vi "Scale.vi"(8 "error in (no error)":errorcluster, 10 "Scale Factor":dbl, 11 "Point in":refnum<class "PointSpecialized.lvclass">) -> (0 "error out":errorcluster, 3 "Point out":refnum<class "PointSpecialized.lvclass">)   [LabVIEW 2021, in "Picture2D.lvlib" / "PointSpecialized.lvclass"]
uses:
  PointSpecialized.lvclass
  PointSpecialized.lvclass/PointSpecialized.ctl
  Pen/Pen.lvclass
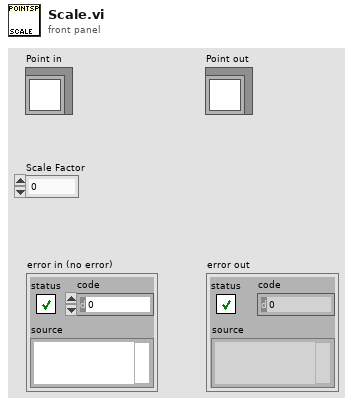
[diagram p1: front panel]
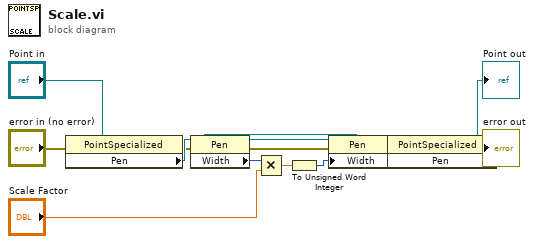
[diagram p0: block diagram]
diagram:
  n1 = property class="PointSpecialized"(reference="Point in", error in="error in (no error)") -> (reference out=w7:refnum<class "PointSpecialized.lvclass">, error out=w5:errorcluster, "Pen"=w15:refnum<class "Pen.lvclass">)
  n2 = property class="Pen"(reference=w15, error in=w5) -> (reference out=w14:refnum<class "Pen.lvclass">, error out=w4:errorcluster, "Width"=w11:u16)
  n3 = Multiply(x=w11, y="Scale Factor") -> (x*y=w10:dbl)
  n4 = To Unsigned Word Integer(number=w10) -> (unsigned 16bit integer=w9:u16)
  n5 = property class="Pen"(reference=w14, error in=w4, "Width"=w9) -> (reference out=w13:refnum<class "Pen.lvclass">, error out=w3:errorcluster)
  n6 = property class="PointSpecialized"(reference=w7, error in=w3, "Pen"=w13) -> (reference out=→"Point out":refnum<class "PointSpecialized.lvclass">, error out=→"error out":errorcluster)
